vi "Trip2_DesiredAngle_noDIO_noAnnotated.vi"(0 "Current Angle":dbl, 2 "X-Position":dbl, 3 "Y-Position":dbl, 8 "Zone A":bool, 9 "Dumping Complete":bool, 10 "Zone B":bool) -> (13 "Commence Mining 2":bool, 14 "RFM":i32, 15 "RMM":i32, 16 "RRM":i32, 17 "LFM":i32, 18 "LMM":i32, 19 "LRM":i32)   [LabVIEW 2014]
panel:
  out "Desired Angle":dbl
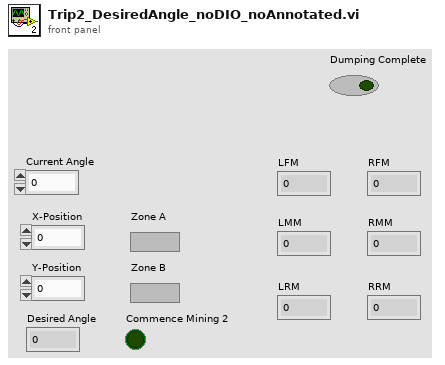
[diagram p1: front panel]
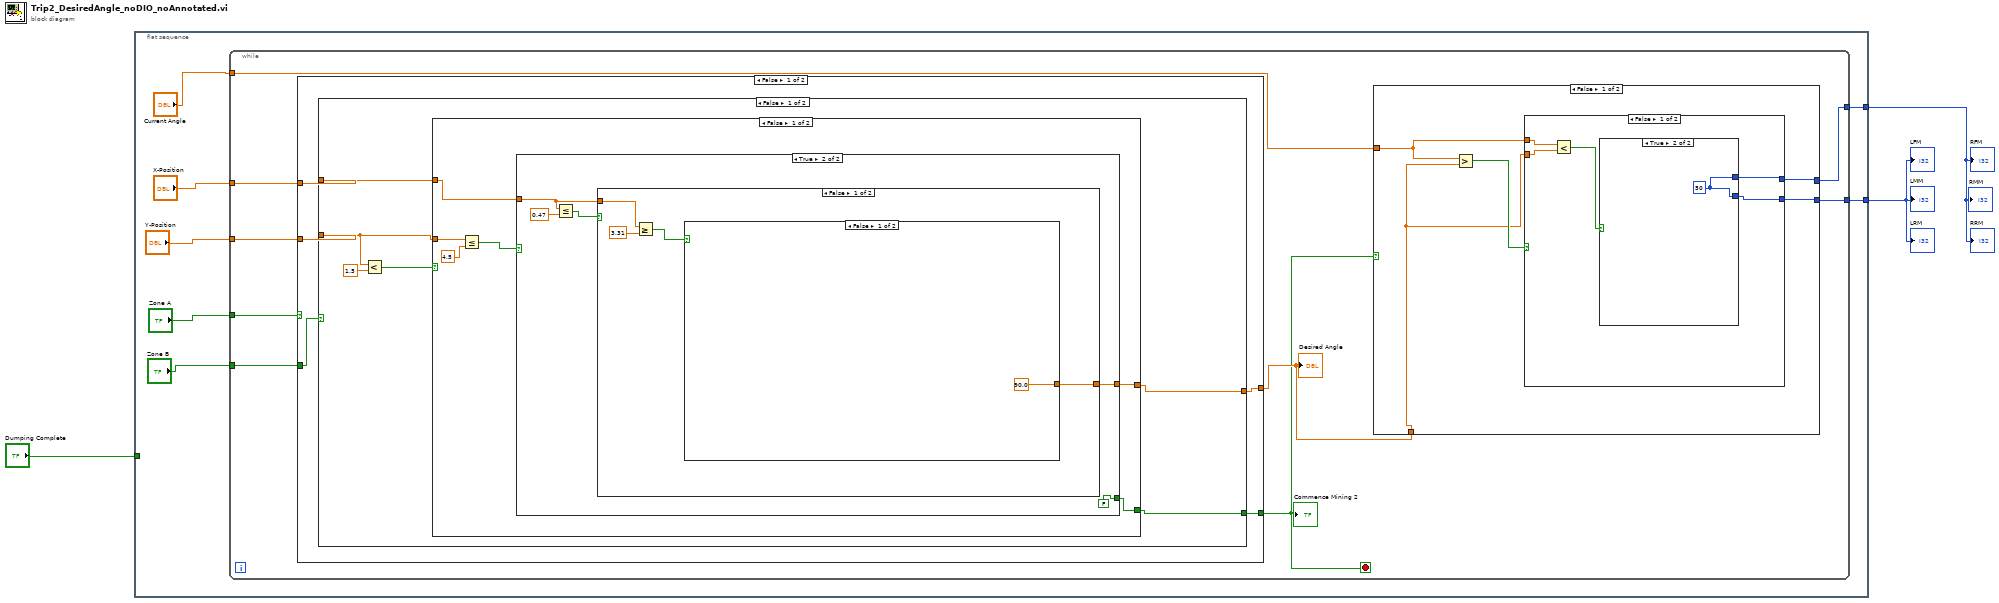
[diagram p0: block diagram]
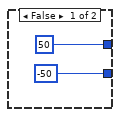
[diagram p2: hidden frame]
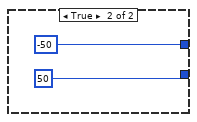
[diagram p3: hidden frame]
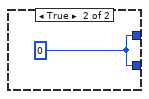
[diagram p4: hidden frame]
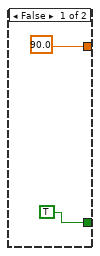
[diagram p5: hidden frame]
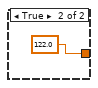
[diagram p6: hidden frame]
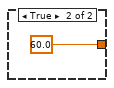
[diagram p7: hidden frame]
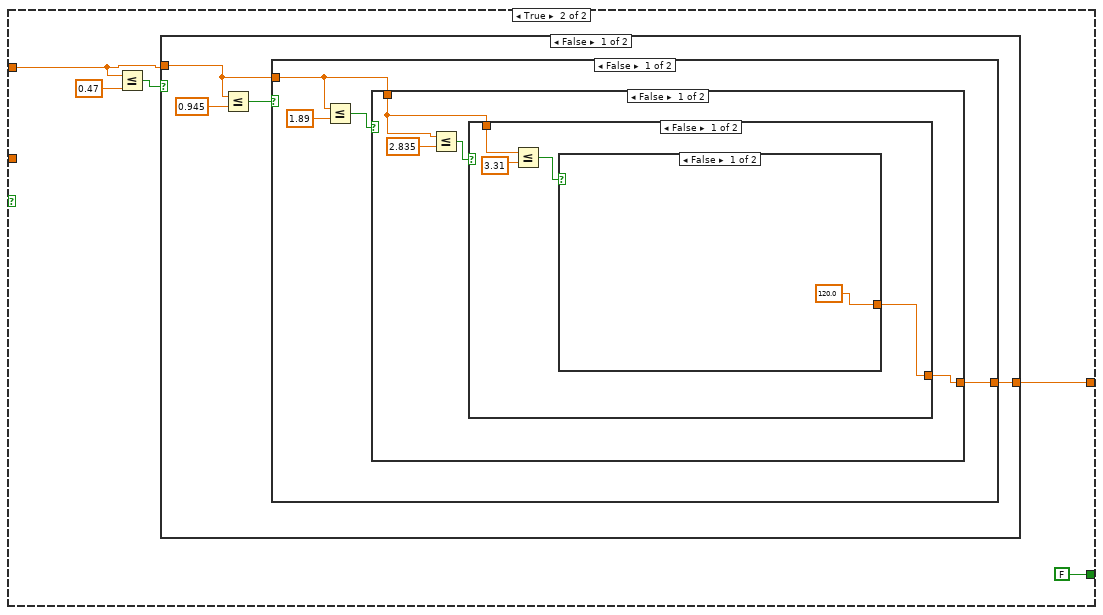
[diagram p8: hidden frame]
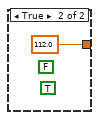
[diagram p9: hidden frame]
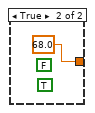
[diagram p10: hidden frame]
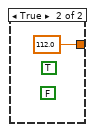
[diagram p11: hidden frame]
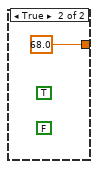
[diagram p12: hidden frame]
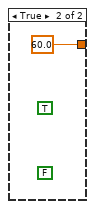
[diagram p13: hidden frame]
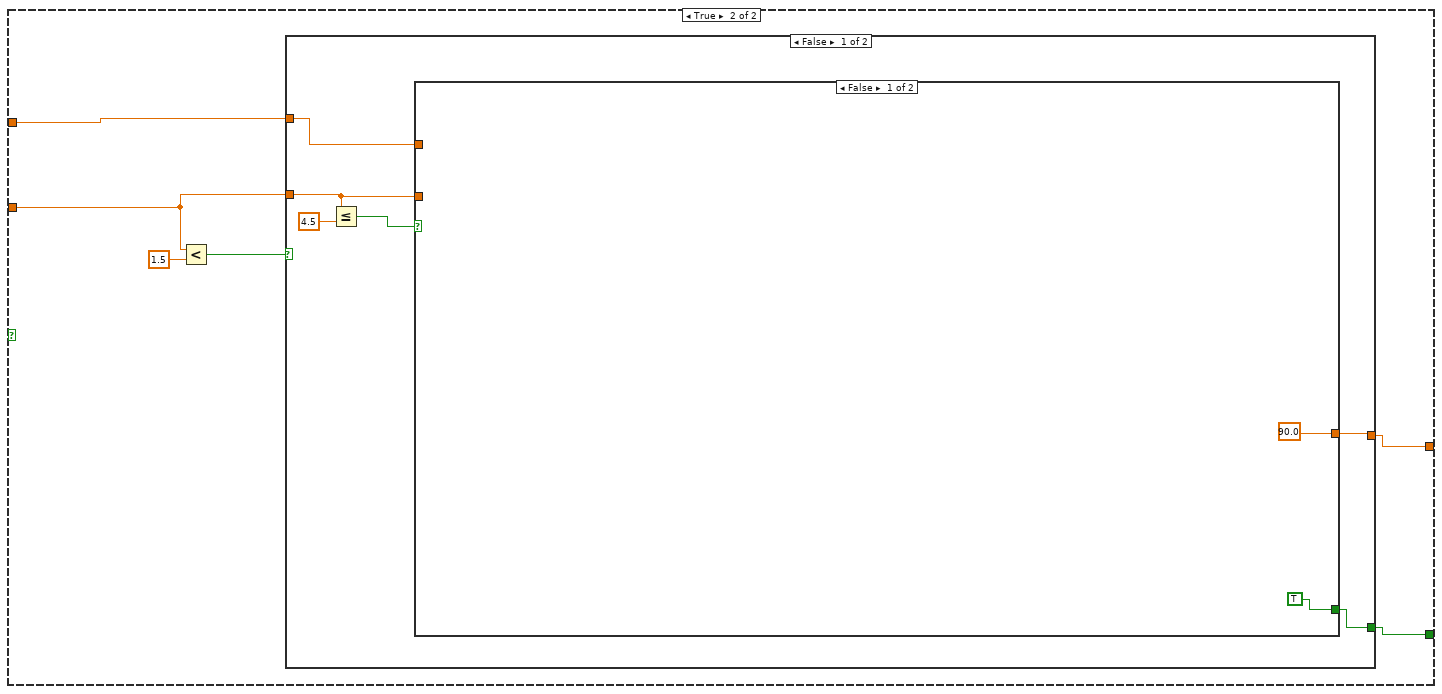
[diagram p14: hidden frame]
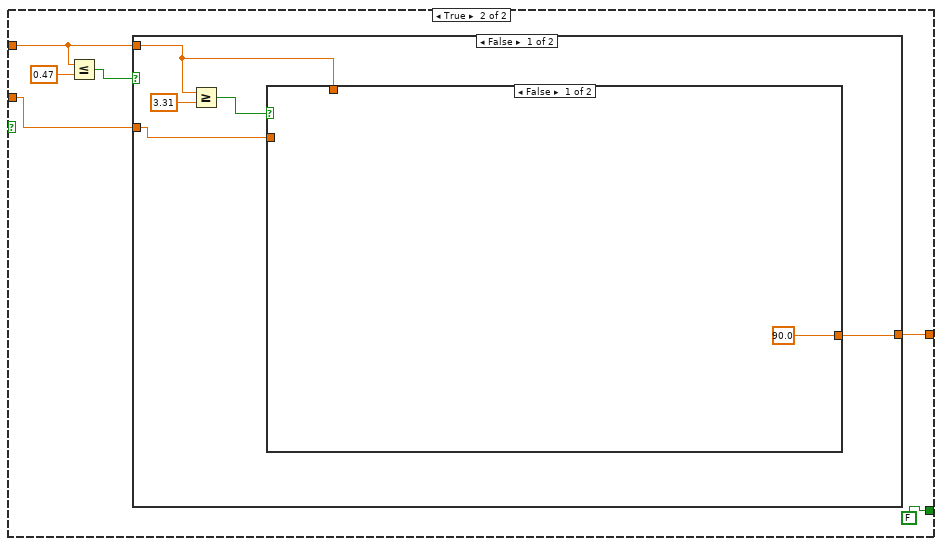
[diagram p15: hidden frame]
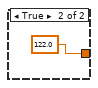
[diagram p16: hidden frame]
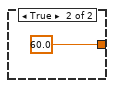
[diagram p17: hidden frame]
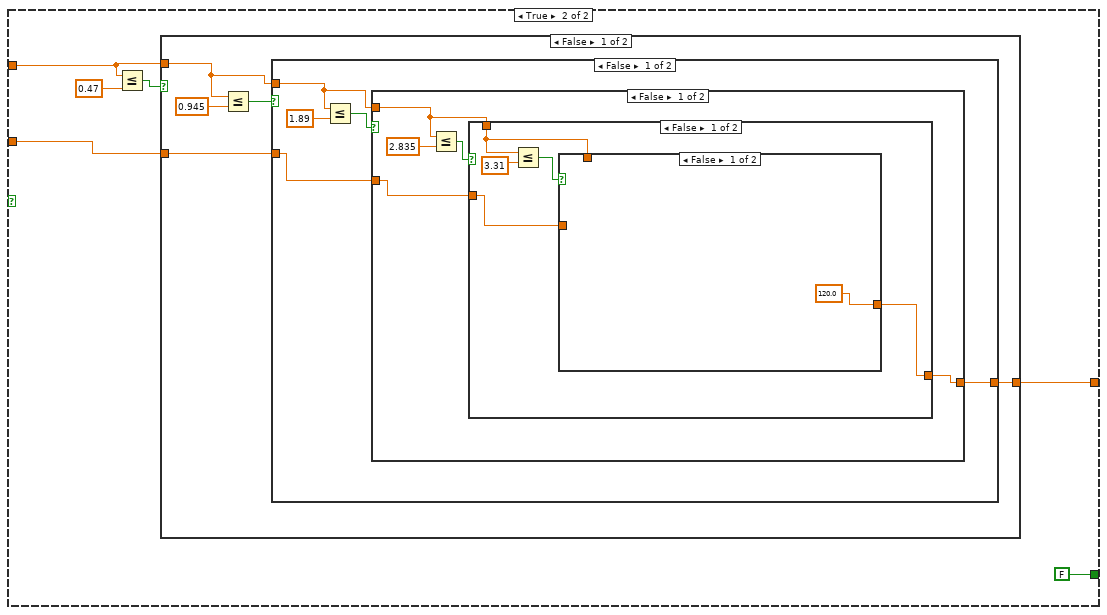
[diagram p18: hidden frame]
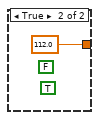
[diagram p19: hidden frame]
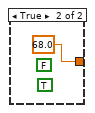
[diagram p20: hidden frame]
diagram:
  n1 = flat-sequence {
    tunnel: [w6] -> w3
    tunnel: [w5] -> w2
    tunnel: "Dumping Complete" -> [_]
    frame #0 {
      n2 = while {
        tunnel: "X-Position" -> [w19]
        tunnel: "Y-Position" -> [w18]
        tunnel: "Zone A" -> [w17]
        tunnel: "Current Angle" -> [w14]
        tunnel: [w13] -> w6
        tunnel: [w12] -> w5
        tunnel: "Zone B" -> [w11]
        stop <- w15 stop-if-true
        n3 = case shown="False" w17 {
          tunnel: [w38 w158] -> w16
          tunnel: w19 -> [w40 w157]
          tunnel: w18 -> [w39 w156]
          tunnel: [w37 w155] -> w15
          tunnel: w11 -> [w36 w154]
          frame False {
            n4 = case shown="False" w36 {
              tunnel: w40 -> [w43 w97]
              tunnel: w39 -> [w44 w96]
              tunnel: [w41 w95] -> w38
              tunnel: [w42 w94] -> w37
              frame False {
                n5 = Less?(x=w44, y=1.5) -> (x < y?=w46:bool)
                n6 = case shown="False" w46 {
                  tunnel: [w52 w71] -> w41
                  tunnel: [w49 FALSE] -> w42
                  tunnel: w44 -> [w48 _]
                  tunnel: w43 -> [w47 w67]
                  frame False {
                    n7 = Less Or Equal?(x=w48, y=4.5) -> (x <= y?=w50:bool)
                    n8 = case shown="True" w50 {
                      tunnel: [90.0 w57] -> w52
                      tunnel: [TRUE FALSE] -> w49
                      tunnel: w47 -> [_ w55]
                      frame False {
                      }
                      frame True {
                        n9 = Less Or Equal?(x=w55, y=0.47) -> (x <= y?=w58:bool)
                        n10 = case shown="False" w58 {
                          tunnel: [w61 60.0] -> w57
                          tunnel: w55 -> [w60 _]
                          frame False {
                            n11 = Greater Or Equal?(x=w60, y=3.31) -> (x >= y?=w62:bool)
                            n12 = case shown="False" w62 {
                              tunnel: [90.0 122.0] -> w61
                              frame False {
                              }
                              frame True {
                              }
                            }
                          }
                          frame True {
                          }
                        }
                      }
                    }
                  }
                  frame True {
                    n13 = Less Or Equal?(x=w67, y=0.47) -> (x <= y?=w69:bool)
                    n14 = case shown="False" w69 {
                      tunnel: [w73 60.0] -> w71
                      tunnel: w67 -> [w72 _]
                      frame False {
                        n15 = Less Or Equal?(x=w72, y=0.945) -> (x <= y?=w75:bool)
                        n16 = case shown="False" w75 {
                          tunnel: [w77 68.0] -> w73
                          tunnel: w72 -> [w76 _]
                          frame False {
                            n17 = Less Or Equal?(x=w76, y=1.89) -> (x <= y?=w78:bool)
                            n18 = case shown="False" w78 {
                              tunnel: [w81 112.0] -> w77
                              tunnel: w76 -> [w80 _]
                              frame False {
                                n19 = Less Or Equal?(x=w80, y=2.835) -> (x <= y?=w82:bool)
                                n20 = case shown="False" w82 {
                                tunnel: [w85 68.0] -> w81
                                tunnel: w80 -> [w84 _]
                                frame False {
                                n21 = Less Or Equal?(x=w84, y=3.31) -> (x <= y?=w86:bool)
                                n22 = case shown="False" w86 {
                                tunnel: [120.0 112.0] -> w85
                                frame False {
                                }
                                frame True {
                                (unwired) TRUE
                                (unwired) FALSE
                                }
                                }
                                }
                                frame True {
                                (unwired) TRUE
                                (unwired) FALSE
                                }
                                }
                              }
                              frame True {
                                (unwired) FALSE
                                (unwired) TRUE
                              }
                            }
                          }
                          frame True {
                            (unwired) FALSE
                            (unwired) TRUE
                          }
                        }
                      }
                      frame True {
                        (unwired) FALSE
                        (unwired) TRUE
                      }
                    }
                  }
                }
              }
              frame True {
                n23 = Less?(x=w96, y=1.5) -> (x < y?=w99:bool)
                n24 = case shown="False" w99 {
                  tunnel: [w105 w127] -> w95
                  tunnel: w97 -> [w104 w125]
                  tunnel: w96 -> [w101 w123]
                  tunnel: [w100 FALSE] -> w94
                  frame False {
                    n25 = Less Or Equal?(x=w101, y=4.5) -> (x <= y?=w102:bool)
                    n26 = case shown="False" w102 {
                      tunnel: [90.0 w111] -> w105
                      tunnel: w104 -> [_ w110]
                      tunnel: w101 -> [_ w109]
                      tunnel: [TRUE FALSE] -> w100
                      frame False {
                      }
                      frame True {
                        n27 = Less Or Equal?(x=w110, y=0.47) -> (x <= y?=w112:bool)
                        n28 = case shown="False" w112 {
                          tunnel: [w116 60.0] -> w111
                          tunnel: w110 -> [w115 _]
                          tunnel: w109 -> [w114 _]
                          frame False {
                            n29 = Greater Or Equal?(x=w115, y=3.31) -> (x >= y?=w117:bool)
                            n30 = case shown="False" w117 {
                              tunnel: [90.0 122.0] -> w116
                              tunnel: w115 -> [_ _]
                              tunnel: w114 -> [_ _]
                              frame False {
                              }
                              frame True {
                              }
                            }
                          }
                          frame True {
                          }
                        }
                      }
                    }
                  }
                  frame True {
                    n31 = Less Or Equal?(x=w125, y=0.47) -> (x <= y?=w124:bool)
                    n32 = case shown="False" w124 {
                      tunnel: w125 -> [w130 _]
                      tunnel: [w129 60.0] -> w127
                      tunnel: w123 -> [w128 _]
                      frame False {
                        n33 = Less Or Equal?(x=w130, y=0.945) -> (x <= y?=w132:bool)
                        n34 = case shown="False" w132 {
                          tunnel: w130 -> [w135 _]
                          tunnel: [w134 68.0] -> w129
                          tunnel: w128 -> [w133 _]
                          frame False {
                            n35 = Less Or Equal?(x=w135, y=1.89) -> (x <= y?=w136:bool)
                            n36 = case shown="False" w136 {
                              tunnel: w135 -> [w140 _]
                              tunnel: [w139 112.0] -> w134
                              tunnel: w133 -> [w138 _]
                              frame False {
                                n37 = Less Or Equal?(x=w140, y=2.835) -> (x <= y?=w141:bool)
                                n38 = case shown="False" w141 {
                                tunnel: w140 -> [w145 _]
                                tunnel: [w144 68.0] -> w139
                                tunnel: w138 -> [w143 _]
                                frame False {
                                n39 = Less Or Equal?(x=w145, y=3.31) -> (x <= y?=w146:bool)
                                n40 = case shown="False" w146 {
                                tunnel: w145 -> [_ _]
                                tunnel: [120.0 112.0] -> w144
                                tunnel: w143 -> [_ _]
                                frame False {
                                }
                                frame True {
                                (unwired) TRUE
                                (unwired) FALSE
                                }
                                }
                                }
                                frame True {
                                (unwired) TRUE
                                (unwired) FALSE
                                }
                                }
                              }
                              frame True {
                                (unwired) FALSE
                                (unwired) TRUE
                              }
                            }
                          }
                          frame True {
                            (unwired) FALSE
                            (unwired) TRUE
                          }
                        }
                      }
                      frame True {
                        (unwired) FALSE
                        (unwired) TRUE
                      }
                    }
                  }
                }
              }
            }
          }
          frame True {
            n41 = case shown="False" w154 {
              tunnel: [w160 w244] -> w158
              tunnel: w157 -> [w162 w243]
              tunnel: w156 -> [w161 w240]
              tunnel: [w159 w239] -> w155
              frame False {
                n42 = Less?(x=w161, y=1.5) -> (x < y?=w163:bool)
                n43 = case shown="False" w163 {
                  tunnel: [w170 w192] -> w160
                  tunnel: w162 -> [w169 w190]
                  tunnel: w161 -> [w166 w188]
                  tunnel: [w165 FALSE] -> w159
                  frame False {
                    n44 = Less Or Equal?(x=w166, y=4.5) -> (x <= y?=w167:bool)
                    n45 = case shown="True" w167 {
                      tunnel: [90.0 w176] -> w170
                      tunnel: w169 -> [_ w175]
                      tunnel: w166 -> [_ w174]
                      tunnel: [TRUE FALSE] -> w165
                      frame False {
                      }
                      frame True {
                        n46 = Less Or Equal?(x=w175, y=0.47) -> (x <= y?=w177:bool)
                        n47 = case shown="False" w177 {
                          tunnel: [w181 60.0] -> w176
                          tunnel: w175 -> [w180 _]
                          tunnel: w174 -> [w179 _]
                          frame False {
                            n48 = Greater Or Equal?(x=w180, y=3.31) -> (x >= y?=w182:bool)
                            n49 = case shown="False" w182 {
                              tunnel: [90.0 122.0] -> w181
                              tunnel: w180 -> [_ _]
                              tunnel: w179 -> [_ _]
                              frame False {
                              }
                              frame True {
                              }
                            }
                          }
                          frame True {
                          }
                        }
                      }
                    }
                  }
                  frame True {
                    n50 = Less Or Equal?(x=w190, y=0.47) -> (x <= y?=w189:bool)
                    n51 = case shown="False" w189 {
                      tunnel: w190 -> [w197 w237]
                      tunnel: [w196 45.0] -> w192
                      tunnel: [w195 w237] -> _
                      tunnel: w188 -> [w194 w236]
                      tunnel: [w193 w236] -> _
                      frame False {
                        n52 = Less Or Equal?(x=w197, y=0.945) -> (x <= y?=w199:bool)
                        n53 = case shown="False" w199 {
                          tunnel: w197 -> [w204 w234]
                          tunnel: [w203 68.0] -> w196
                          tunnel: [w202 w234] -> w195
                          tunnel: w194 -> [w201 w233]
                          tunnel: [w200 w233] -> w193
                          frame False {
                            n54 = Less Or Equal?(x=w204, y=1.89) -> (x <= y?=w205:bool)
                            n55 = case shown="True" w205 {
                              tunnel: w204 -> [w211 w231]
                              tunnel: [w210 112.0] -> w203
                              tunnel: [w209 w231] -> w202
                              tunnel: w201 -> [w208 w230]
                              tunnel: [w207 w230] -> w200
                              frame False {
                                n56 = Less Or Equal?(x=w211, y=2.835) -> (x <= y?=w212:bool)
                                n57 = case shown="False" w212 {
                                tunnel: w211 -> [w218 w228]
                                tunnel: [w217 68.0] -> w210
                                tunnel: [w216 w228] -> w209
                                tunnel: w208 -> [w215 w227]
                                tunnel: [w214 w227] -> w207
                                frame False {
                                n58 = Less Or Equal?(x=w218, y=3.31) -> (x <= y?=w219:bool)
                                n59 = case shown="False" w219 {
                                tunnel: w218 -> [w222 w225]
                                tunnel: [120.0 112.0] -> w217
                                tunnel: [w222 w225] -> w216
                                tunnel: w215 -> [w221 w224]
                                tunnel: [w221 w224] -> w214
                                frame False {
                                }
                                frame True {
                                (unwired) TRUE
                                (unwired) FALSE
                                }
                                }
                                }
                                frame True {
                                (unwired) TRUE
                                (unwired) FALSE
                                }
                                }
                              }
                              frame True {
                              }
                            }
                          }
                          frame True {
                            (unwired) FALSE
                            (unwired) TRUE
                          }
                        }
                      }
                      frame True {
                      }
                    }
                  }
                }
              }
              frame True {
                n60 = Less?(x=w240, y=1.5) -> (x < y?=w241:bool)
                n61 = case shown="False" w241 {
                  tunnel: [w250 w280] -> w244
                  tunnel: w243 -> [w249 w278]
                  tunnel: w240 -> [w246 w276]
                  tunnel: [w245 FALSE] -> w239
                  frame False {
                    n62 = Less Or Equal?(x=w246, y=4.5) -> (x <= y?=w247:bool)
                    n63 = case shown="False" w247 {
                      tunnel: [90.0 w256] -> w250
                      tunnel: w249 -> [_ w255]
                      tunnel: w246 -> [_ w254]
                      tunnel: [TRUE FALSE] -> w245
                      frame False {
                      }
                      frame True {
                        n64 = Less Or Equal?(x=w255, y=0.47) -> (x <= y?=w257:bool)
                        n65 = case shown="False" w257 {
                          tunnel: [w263 60.0] -> w256
                          tunnel: w255 -> [w262 w273]
                          tunnel: w254 -> [w261 w272]
                          tunnel: [w260 w272] -> _
                          tunnel: [w259 w273] -> _
                          frame False {
                            n66 = Greater Or Equal?(x=w262, y=3.31) -> (x >= y?=w264:bool)
                            n67 = case shown="False" w264 {
                              tunnel: [90.0 122.0] -> w263
                              tunnel: w262 -> [w266 w270]
                              tunnel: w261 -> [w267 w269]
                              tunnel: [w267 w269] -> w260
                              tunnel: [w266 w270] -> w259
                              frame False {
                              }
                              frame True {
                              }
                            }
                          }
                          frame True {
                          }
                        }
                      }
                    }
                  }
                  frame True {
                    n68 = Less Or Equal?(x=w278, y=0.47) -> (x <= y?=w277:bool)
                    n69 = case shown="False" w277 {
                      tunnel: w278 -> [w283 _]
                      tunnel: [w282 60.0] -> w280
                      tunnel: w276 -> [w281 _]
                      frame False {
                        n70 = Less Or Equal?(x=w283, y=0.945) -> (x <= y?=w285:bool)
                        n71 = case shown="False" w285 {
                          tunnel: w283 -> [w288 _]
                          tunnel: [w287 68.0] -> w282
                          tunnel: w281 -> [w286 _]
                          frame False {
                            n72 = Less Or Equal?(x=w288, y=1.89) -> (x <= y?=w289:bool)
                            n73 = case shown="False" w289 {
                              tunnel: w288 -> [w293 _]
                              tunnel: [w292 112.0] -> w287
                              tunnel: w286 -> [w291 _]
                              frame False {
                                n74 = Less Or Equal?(x=w293, y=2.835) -> (x <= y?=w294:bool)
                                n75 = case shown="False" w294 {
                                tunnel: w293 -> [w298 _]
                                tunnel: [w297 68.0] -> w292
                                tunnel: w291 -> [w296 _]
                                frame False {
                                n76 = Less Or Equal?(x=w298, y=3.31) -> (x <= y?=w299:bool)
                                n77 = case shown="False" w299 {
                                tunnel: w298 -> [_ _]
                                tunnel: [120.0 112.0] -> w297
                                tunnel: w296 -> [_ _]
                                frame False {
                                }
                                frame True {
                                (unwired) TRUE
                                (unwired) FALSE
                                }
                                }
                                }
                                frame True {
                                (unwired) TRUE
                                (unwired) FALSE
                                }
                                }
                              }
                              frame True {
                                (unwired) FALSE
                                (unwired) TRUE
                              }
                            }
                          }
                          frame True {
                            (unwired) FALSE
                            (unwired) TRUE
                          }
                        }
                      }
                      frame True {
                        (unwired) FALSE
                        (unwired) TRUE
                      }
                    }
                  }
                }
              }
            }
          }
        }
        "Commence Mining 2" <- w15
        "Desired Angle" <- w16
        n78 = case shown="False" w15 {
          tunnel: w14 -> [w23 _]
          tunnel: w16 -> [w22 _]
          tunnel: [w20 w35] -> w13
          tunnel: [w21 w35] -> w12
          frame False {
            n79 = Greater?(x=w23, y=w22) -> (0:w24:bool)
            n80 = case shown="False" w24 {
              tunnel: w23 -> [w29 _]
              tunnel: w22 -> [w28 _]
              tunnel: [w26 -50] -> w21
              tunnel: [w25 50] -> w20
              frame False {
                n81 = Less?(x=w29, y=w28) -> (x < y?=w27:bool)
                n82 = case shown="True" w27 {
                  tunnel: [50 w32] -> w26
                  tunnel: [-50 w32] -> w25
                  frame False {
                  }
                  frame True {
                    w32 = 50
                  }
                }
              }
              frame True {
              }
            }
          }
          frame True {
            w35 = 0
          }
        }
      }
    }
  }
  "RFM" <- w2
  "RMM" <- w2
  "RRM" <- w2
  "LFM" <- w3
  "LMM" <- w3
  "LRM" <- w3
